vi "pattern.vi"() -> ()   [LabVIEW 2025]
uses:
  <instrlib>/Chrome 19025/Chrome 19025.lvlib
  Type Def/steps--numeric.ctl
panel:
  out "error out":errorcluster
  in  "error in (no error)":errorcluster
  out "VISA resource name out":refnum<visa-resource-name>
  in  "VISA resource name":refnum<visa-resource-name>
  out "Result":string
  in  "Step":T1=1 min=1 max=99 step=1
  # "query"
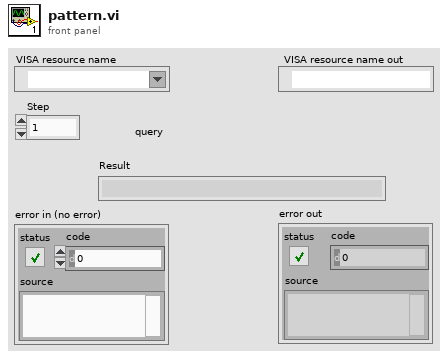
[diagram p1: front panel]
types:
  T1 = typedef "steps--numeric.ctl" = u8
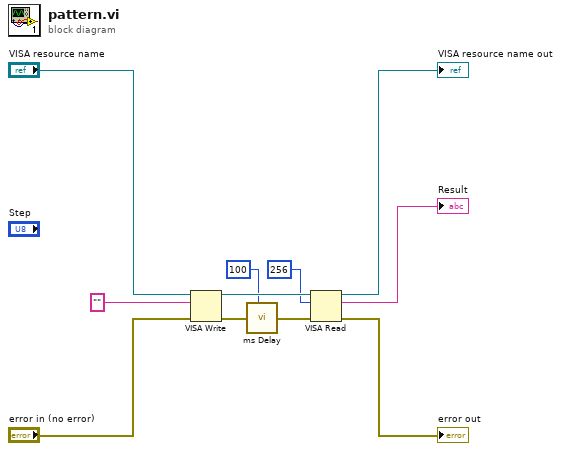
[diagram p0: block diagram]
diagram:
  n1 = VISA Write(VISA resource name="VISA resource name", write buffer="", error in (no error)="error in (no error)") -> (VISA resource name out=w11:refnum<visa-resource-name>, error out=w10:errorcluster)  [unwired: 1 out]
  n2 = call <instrlib>:"ms Delay.vi"("miliseconds to wait"=u32 100 ("Time Delay ms"), "error in (no error)"=w10) -> ("error out"=w9:errorcluster)  [unwired: 6 in, 1 out]
  n3 = VISA Read(VISA resource name=w11, byte count=u32 256, error in (no error)=w9) -> (VISA resource name out=→"VISA resource name out":refnum<visa-resource-name>, read buffer=→"Result":string, error out=→"error out":errorcluster)  [unwired: 1 out]
